vi "line_counter_for_z_steps.vi"(1 "lines per z step":u16, 2 "line counter for z steps":u16, 3 "end of line?":bool) -> (0 "line counter for z steps out":u16)   [LabVIEW 2010]
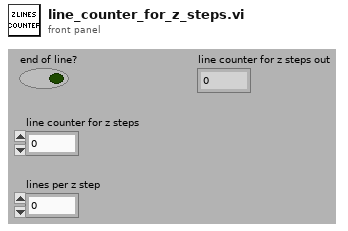
[diagram p1: front panel]
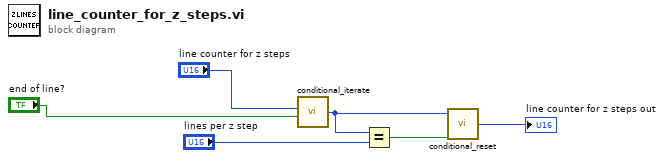
[diagram p0: block diagram]
diagram:
  n1 = call "conditional_iterate.vi"("iterate?"="end of line?", "number in"="line counter for z steps") -> ("number out"=w5:u16)  [unwired: 4 in]
  n2 = Equal?(x=w5, y="lines per z step") -> (x = y?=w4:bool)
  n3 = call "conditional_reset.vi"("reset?"=w4, "number in"=w5) -> ("number out"=→"line counter for z steps out":u16)  [unwired: 4 in]
